vi "Database_to_string.vi"(8 "error in (no error)":errorcluster, 11 "Array":T1[](array[typedef])) -> (0 "error out":errorcluster, 3 "String":string)   [LabVIEW 2022 SP3]
uses:
  Database_element.ctl
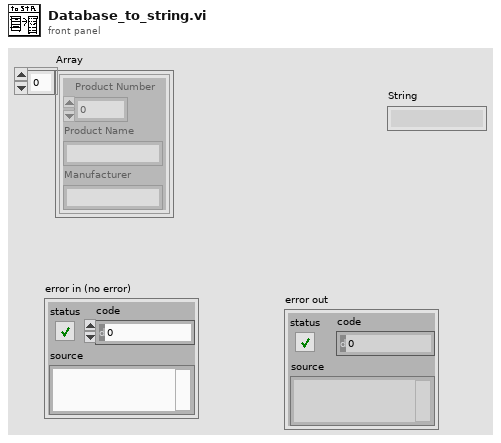
[diagram p1: front panel]
types:
  T1 = typedef "Database_element.ctl" = cluster{"Product Number":i32, "Product Name":string, "Manufacturer":string}
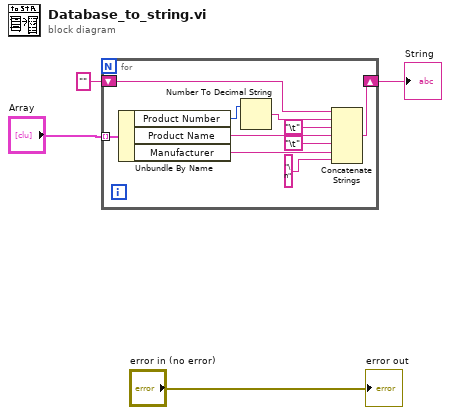
[diagram p0: block diagram]
diagram:
  n1 = for {
    tunnel: "Array" -> [w14] mode=indexing
    shift-right: [w6] -> w1
    shift-left: "" -> [w5]
    n2 = Unbundle By Name(w14) -> ("Product Number"=w13:i32, "Product Name"=w11:string, "Manufacturer"=w10:string)
    n3 = Number To Decimal String(number=w13) -> (decimal integer string=w12:string)  [unwired: 1 in]
    n4 = Concatenate Strings(w5, w12, "\t", w11, "\t", w10, "\n" ("string")) -> (w6:string)
  }
  "String" <- w1
  "error out" <- "error in (no error)"
